vi "#PCBs on panel.vi"(8 "error in (no error)":errorcluster) -> (0 "error out":errorcluster, 3 "# PCBS on Panel out":u32)   [LabVIEW 2013, in "Manipulate IPF.lvlib"]
uses:
  Manipulate IPF.lvlib
  a3Di APG.lvlib
panel:
  in  "#  PCBS on Panel":u32=1 min=1 step=1
  in  "OK":bool
  # "#  PCBs on Panel"
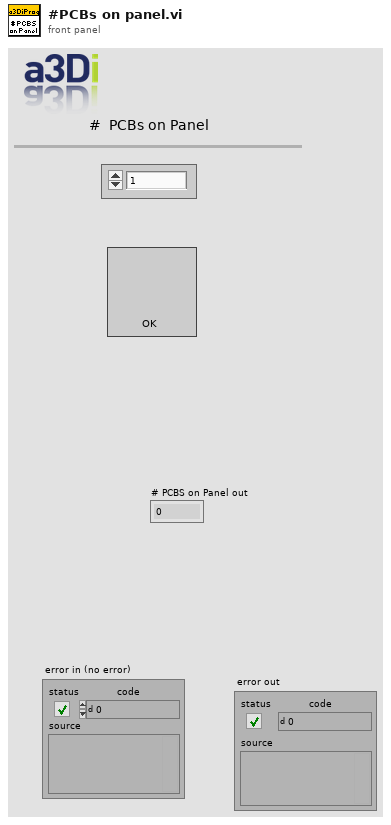
[diagram p1: front panel]
types:
  T1 = enum32{"Invalid", "Standard", "Closed", "Hidden", "Minimized", "Maximized"}
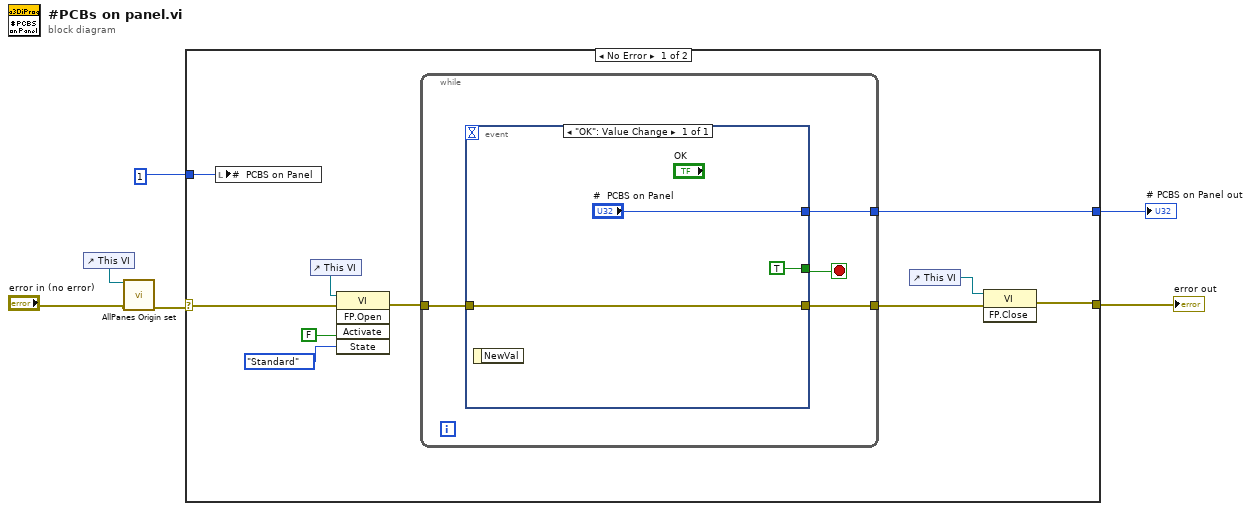
[diagram p0: block diagram]
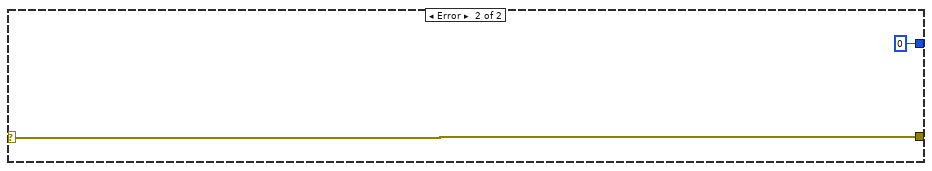
[diagram p2: hidden frame]
diagram:
  n1 = control-ref of="This VI"() -> (w1:refnum<vi>)
  n2 = call "AllPanes Origin set.vi"("VI ref in"=w1, "error in"="error in (no error)") -> ("error out"=w2:errorcluster)  [unwired: 12 in, 1 out]
  n3 = case shown="No Error" w2 {
    selector: w2 -> [w10 w25]
    tunnel: [w11 w25] -> w6
    tunnel: [w9 u32 0 ("#  PCBS on Panel")] -> w5
    tunnel: u32 1 ("#  PCBS on Panel") -> [w7 _]
    frame No Error {
      n4 = local write "#  PCBS on Panel"(w7) -> ()
      n5 = control-ref of="This VI"() -> (w16:refnum<vi>)
      n6 = invoke class="VI" method="FP.Open"(reference=w16, error in=w10, "Activate"=FALSE ("Activate?"), "State"=T1."Standard") -> (error out=w13:errorcluster)  [unwired: 1 in, 4 out]
      n7 = while {
        tunnel: w13 -> [w20]
        tunnel: [w19] -> w9
        tunnel: [w17] -> w8
        stop <- w18 stop-if-true
        n8 = event shown="[0] \"OK\": Value Change" {
          selector: _ -> [_]
          dyn-events: _ -> [_]
          timeout: _ -> [_]
          tunnel: w20 -> [w22]
          tunnel: [w22] -> w17
          tunnel: [TRUE] -> w18
          tunnel: ["#  PCBS on Panel"] -> w19
          event "OK": Value Change {
            n9 = event-data() -> ()  [unwired: 1 in, 1 out]
          }
        }
      }
      n10 = control-ref of="This VI"() -> (w12:refnum<vi>)
      n11 = invoke class="VI" method="FP.Close"(reference=w12, error in=w8) -> (error out=w11:errorcluster)  [unwired: 1 in, 2 out]
    }
    frame Error {
    }
  }
  "error out" <- w6
  "# PCBS on Panel out" <- w5
